vi "joystick deadband.vi"(4 "Joystick In":dbl, 5 "Deadband Range":cluster{"Deadband Min":dbl, "Deadband Max":dbl}={"Deadband Min"=-0.05, "Deadband Max"=0.05}) -> (1 "Joystick Out":dbl)   [LabVIEW 2014]
doc: "This VI will replace numbers between the Min and Max parameters with zero. Useful for applying a deadband on a joystick."
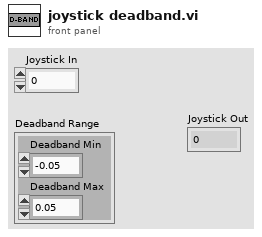
[diagram p1: front panel]
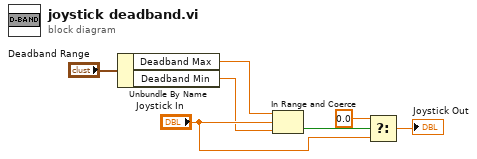
[diagram p0: block diagram]
diagram:
  n1 = Unbundle By Name("Deadband Range") -> ("Deadband Max"=w1:dbl, "Deadband Min"=w2:dbl)
  n2 = In Range and Coerce(upper limit=w1, x="Joystick In", lower limit=w2) -> (In Range?=w7:bool)  [unwired: 1 out]
  n3 = Select(t=0.0, s=w7, f="Joystick In") -> (s? t:f=→"Joystick Out":dbl)
